vi "HostDataGLOBAL (1).vi"() -> ()   [LabVIEW 2017]
panel:
  out "Labels":string[](array[string])
  in  "Data":dbl[](array[numeric])
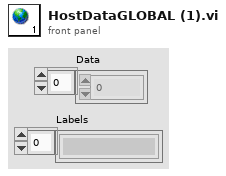
[diagram p1: front panel]
diagram:
